vi "Inficon Units.vi"(8 "Error In":errorcluster, 11 "Emerson Flow Meter Data Input":T1) -> (0 "Error Out":errorcluster, 1 "Basic Units":string[](array[string]), 2 "Units with Mean, STD, ect":string[](array[string]), 3 "Emerson Flow Meter Data Output":T1)   [LabVIEW 2019]
uses:
  Type Definitions/Inficon Data.ctl
panel:
  # "Natural Gas"
  # "Propane"
  # "Natural Gas"
  # "Propane"
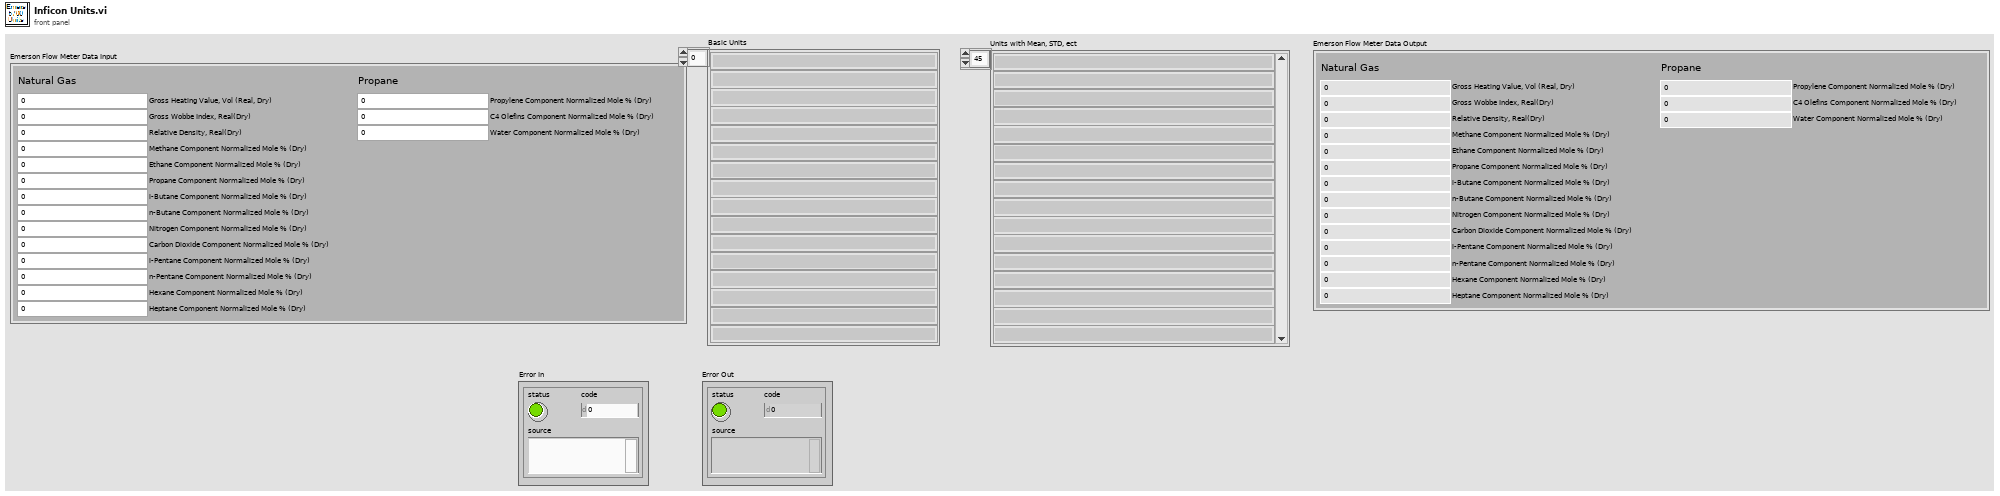
[diagram p1: front panel]
types:
  T1 = typedef "Inficon Data.ctl" = cluster{"Gross Heating Value, Vol (Real, Dry)":dbl, "Nitrogen Component Normalized Mole % (Dry)":dbl, "Methane Component Normalized Mole % (Dry)":dbl, "Carbon Dioxide Component Normalized Mole % (Dry)":dbl, "Ethane Component Normalized Mole % (Dry)":dbl, "Propane Component Normalized Mole % (Dry)":dbl, "i-Pentane Component Normalized Mole % (Dry)":dbl, "i-Butane Component Normalized Mole % (Dry)":dbl, "n-Butane Component Normalized Mole % (Dry)":dbl, "n-Pentane Component Normalized Mole % (Dry)":dbl, "Hexane Component Normalized Mole % (Dry)":dbl, "Heptane Component Normalized Mole % (Dry)":dbl, "Gross Wobbe Index, Real(Dry)":dbl, "Relative Density, Real(Dry)":dbl, "Propylene Component Normalized Mole % (Dry)":dbl, "C4 Olefins Component Normalized Mole % (Dry)":dbl, "Water Component Normalized Mole % (Dry)":dbl}
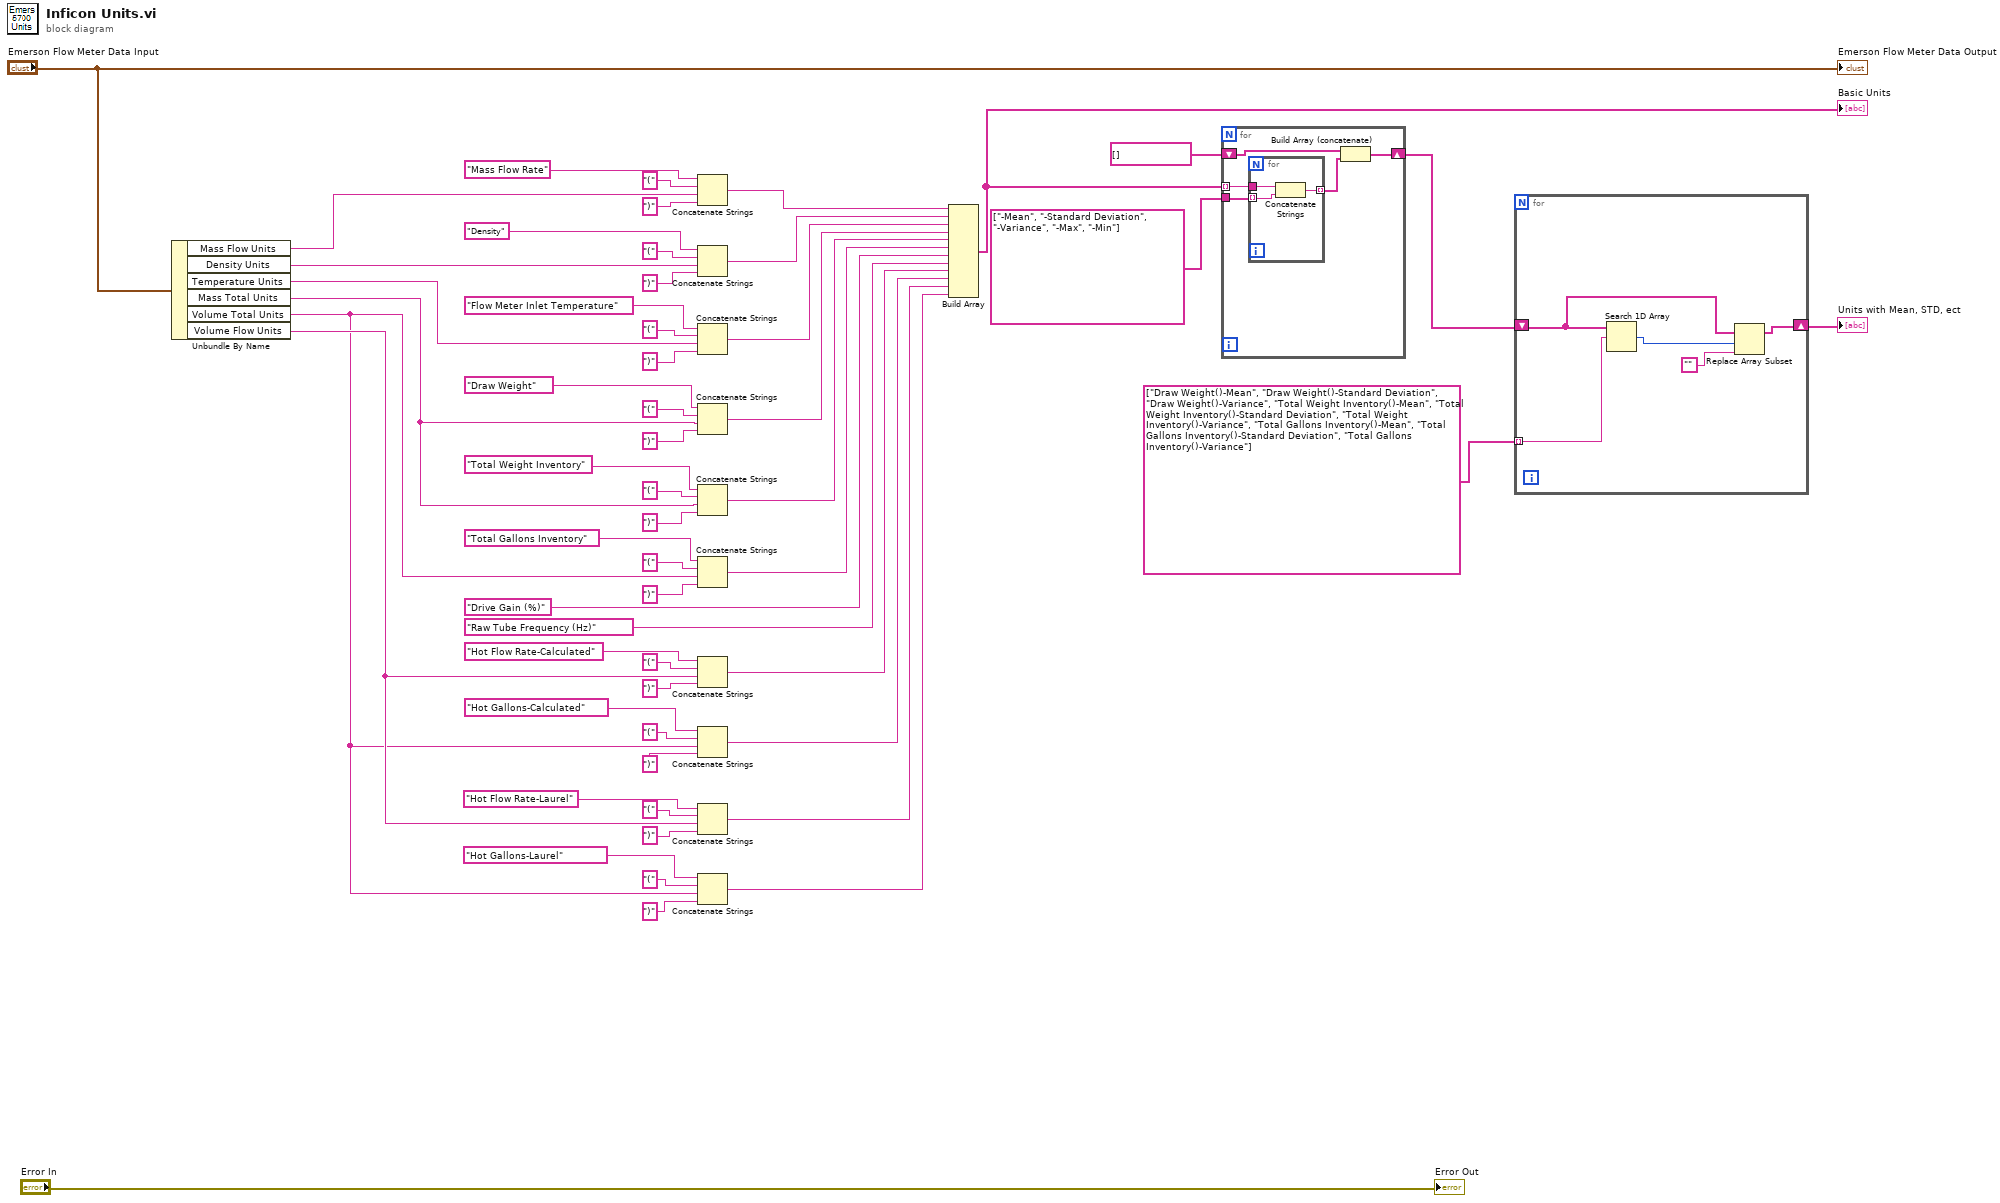
[diagram p0: block diagram]
diagram:
  n1 = Unbundle By Name("Emerson Flow Meter Data Input") -> ("Mass Flow Units"=w53:string, "Density Units"=w54:string, "Temperature Units"=w55:string, "Mass Total Units"=w56:string, "Volume Total Units"=w3:string, "Volume Flow Units"=w4:string)
  n2 = Concatenate Strings("Mass Flow Rate", "(" ("string"), w53, ")" ("string")) -> (w44:string)
  n3 = Concatenate Strings("Density", "(" ("string"), w54, ")" ("string")) -> (w45:string)
  n4 = Concatenate Strings("Flow Meter Inlet Temperature", "(" ("string"), w55, ")" ("string")) -> (w46:string)
  n5 = Concatenate Strings("Draw Weight", "(" ("string"), w56, ")" ("string")) -> (w47:string)
  n6 = Concatenate Strings("Total Weight Inventory", "(" ("string"), w56, ")" ("string")) -> (w48:string)
  n7 = Concatenate Strings("Total Gallons Inventory", "(" ("string"), w3, ")" ("string")) -> (w49:string)
  n8 = Concatenate Strings("Hot Flow Rate-Calculated", "(" ("string"), w4, ")" ("string")) -> (w12:string)
  n9 = Concatenate Strings("Hot Gallons-Calculated", "(" ("string"), w3, ")" ("string")) -> (w11:string)
  n10 = Concatenate Strings("Hot Flow Rate-Laurel", "(" ("string"), w4, ")" ("string")) -> (w2:string)
  n11 = Concatenate Strings("Hot Gallons-Laurel", "(" ("string"), w3, ")" ("string")) -> (w1:string)
  n12 = Build Array(w44, w45, w46, w47, w48, w49, "Drive Gain (%)", "Raw Tube Frequency (Hz)", w12, w11, w2, w1) -> (w25:string[])
  "Basic Units" <- w25
  n13 = for {
    tunnel: w25 -> [w61] mode=indexing
    tunnel: string[] ["-Mean", "-Standard Deviation", "-Variance", "-Max", "-Min"] -> [w60]
    shift-right: [w57] -> w21
    shift-left: string[] [] -> [w59]
    n14 = for {
      tunnel: w61 -> [w64]
      tunnel: w60 -> [w63] mode=indexing
      tunnel: [w62] -> w58 mode=indexing
      n15 = Concatenate Strings(w64, w63) -> (w62:string)
    }
    n16 = Build Array (concatenate)(w59, w58) -> (w57:string[])
  }
  n17 = for {
    tunnel: string[] ["Draw Weight()-Mean", "Draw Weight()-Standard Deviation", "Draw Weight()-Variance", "Total Weight Inventory()-Mean", "Total Weight Inventory()-Standard Deviation", "Total Weight Inventory()-Variance", "Total Gallons Inventory()-Mean", "Total Gallons Inventory()-Standard Deviation", "Total Gallons Inventory()-Variance"] -> [w69] mode=indexing
    shift-right: [w65] -> w19
    shift-left: w21 -> [w68]
    n18 = Search 1D Array(1D array=w68, element=w69) -> (index of element=w67:i32)  [unwired: 1 in]
    n19 = Replace Array Subset(array=w68, new element="", index=w67) -> (w65:string[])
  }
  "Units with Mean, STD, ect" <- w19
  "Error Out" <- "Error In"
  "Emerson Flow Meter Data Output" <- "Emerson Flow Meter Data Input"
